vi "GetDevices.vi"() -> ()   [LabVIEW 2018]
panel:
  out "data out":string
  in  "data in":string="SAY_HELLO_WOLRD"
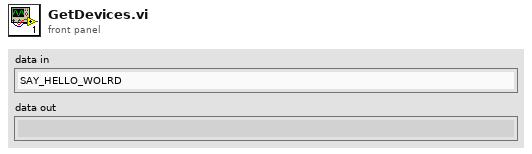
[diagram p1: front panel]
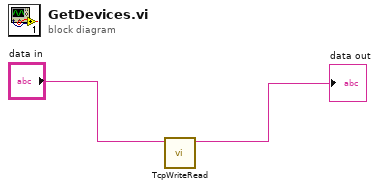
[diagram p0: block diagram]
diagram:
  n1 = call "TcpWriteRead.vi"("data in"="data in") -> ("data out"=→"data out":string)  [unwired: 9 in, 1 out]
